vi "DEV connect to DB and get some data.vi"() -> ()   [LabVIEW 2018, in "Database.lvlib"]
uses:
  <vilib>/addons/database/Connection.llb/DB Tools Open Connec (Path).vi
  Database.lvlib
  <vilib>/addons/database/NI_Database_API.lvlib
panel:
  out "tables":string[](array[string])
  out "data":variant[][](array[variant])
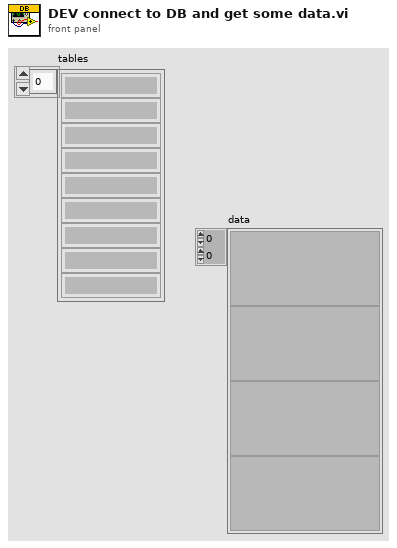
[diagram p1: front panel]
types:
  T1 = typedef "NI_Database_API.lvlib/Conn ObjectReference.ctl" = refnum<k1>
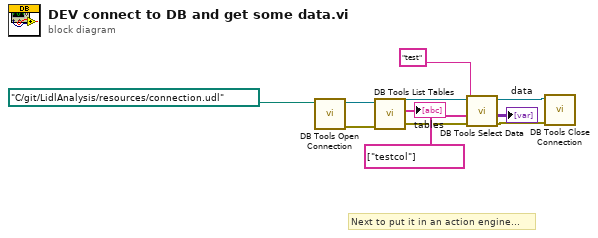
[diagram p0: block diagram]
diagram:
  # "Next to put it in an action engine..."
  n1 = call-poly <vilib>:"DB Tools Open Connection.vi"("connection information"=path "C:/git/LidlAnalysis/resources/connection.udl") -> ("error out"=w10:errorcluster, "connection reference"=w9:T1)  [unwired: 7 in]
  n2 = call <vilib>:"DB Tools List Tables.vi"("error in (no error)"=w10, "connection reference"=w9) -> ("error out"=w6:errorcluster, "tables"=→"tables":string[], "connection reference out"=w5:T1)  [unwired: 3 in]
  n3 = call <vilib>:"DB Tools Select Data.vi"("error in (no error)"=w6, "columns"=string[] ["testcol"], "table"="test", "connection reference"=w5) -> ("error out"=w3:errorcluster, "data"=→"data":variant[][], "connection reference out"=w4:T1)  [unwired: 2 in]
  n4 = call <vilib>:"DB Tools Close Connection.vi"("error in (no error)"=w3, "connection reference"=w4) -> ()  [unwired: 5 in, 1 out]
